vi "Overlay.vi"(8 "error in (no error)":errorcluster, 10 "Image In":T1, 11 "Overlay Base in":refnum<class "Analyze Results SHG-AK.lvclass">) -> (0 "error out":errorcluster, 2 "Image out":T1, 3 "Overlay Base out":refnum<class "Analyze Results SHG-AK.lvclass">)   [LabVIEW 2020, in "Analyze Results SHG-AK.lvclass"]
uses:
  Analyze Results SHG-AK.lvclass
  C:/POLARIS Programme/POLARIS-AS-3-Cams/Submodules/HIJ Vision/Analyze/Results and Overlays/Results Base/Analyze Results Base.lvclass
  <vilib>/vision/Image Controls.llb/IMAQ Image.ctl
  Results Base/Analyze Results Base.lvclass/Analyze Results Base.ctl
  Analyze Results SHG-AK.lvclass/Analyze Results SHG-AK.ctl
  Results Base/Read Overlay_.vi
  Results Base/Read Overlay colors.vi
  Results Base/Read Font, Size & Style.vi
  Results Base/Read Position.vi
  Read FWHM .vi
  Read FWHM Gaussfit.vi
  Results Base/Analyze Results Base.lvclass
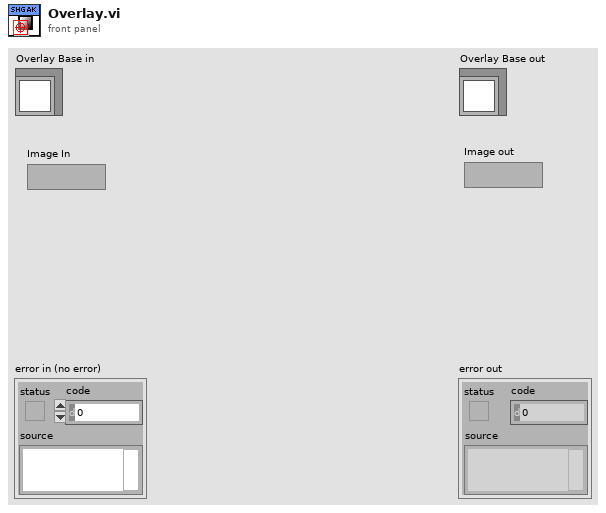
[diagram p1: front panel]
types:
  T1 = typedef "IMAQ Image.ctl" = refnum<image>
  T2 = cluster{"Desired Font (Application)":enum16{"User-specified Font", "Application Font", "System Font", "Dialog Font"}, "[User-specified Font]":cluster{"Font Name":string, "Size":i16, "Strikeout?":bool, "Italic?":bool, "Underline?":bool, "Outline?":bool, "Shadow?":bool, "Bold?":bool, "Rotation Angle":dbl}, "Horizontal Alignment":i16, "Vertical Alignment":i16}
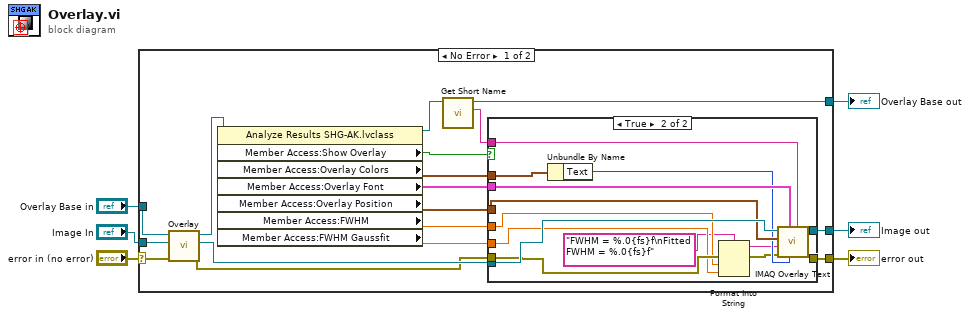
[diagram p0: block diagram]
diagram:
  n1 = case shown="No Error" "error in (no error)" {
    selector: "error in (no error)" -> [w10 w42]
    tunnel: "Image In" -> [w22 w41]
    tunnel: "Overlay Base in" -> [w21 w40]
    tunnel: [w8 w40] -> w4
    tunnel: [w17 w41] -> w3
    tunnel: [w16 w42] -> w2
    frame No Error {
      n2 = call-parent "Overlay.vi"("error in (no error)"=w10, "Image In"=w22, "Overlay Base in"=w21) -> ("error out"=w15:errorcluster, "Image out"=w18:T1, "Overlay Base out"=w23:refnum<class "Analyze Results SHG-AK.lvclass">)  [unwired: 6 in]
      n3 = property class="Analyze Results SHG-AK.lvclass"(reference=w23) -> (reference out=w20:refnum<class "Analyze Results SHG-AK.lvclass">, "Member Access:Show Overlay"=w9:bool, "Member Access:Overlay Colors"=w19:cluster{"Border":u32, "Text":u32}, "Member Access:Overlay Font"=w11:T2, "Member Access:Overlay Position"=w14:cluster{"x":i16, "y":i16}, "Member Access:FWHM "=w13:dbl[unit], "Member Access:FWHM Gaussfit"=w12:dbl[unit])  [unwired: 1 in, 1 out]
      n4 = call-dynamic "Get Short Name.vi"("Analyze Results Base in"=w20) -> ("Short Name"=w7:string, "Analyze Results Base out"=w8:refnum<class "Analyze Results SHG-AK.lvclass">)  [unwired: 8 in, 1 out]
      n5 = case shown="True" w9 {
        tunnel: w19 -> [_ w39]
        tunnel: w18 -> [w25 w38]
        tunnel: [w25 w37] -> w17
        tunnel: [w24 w36] -> w16
        tunnel: w15 -> [w24 w35]
        tunnel: w14 -> [_ w34]
        tunnel: w13 -> [_ w33]
        tunnel: w12 -> [_ w32]
        tunnel: w11 -> [_ w31]
        tunnel: w7 -> [_ w30]
        frame False {
        }
        frame True {
          n6 = Unbundle By Name(w39) -> ("Text"=w29:u32)
          n7 = Format Into String(format string="FWHM = %.0{fs}f\nFitted FWHM = %.0{fs}f", error in=w35, w33, w32) -> (resulting string=w28:string, error out=w27:errorcluster)  [unwired: 1 in]
          n8 = call "IMAQ Overlay Text"("Group"=w30, "Text Color (black)"=w29, "Font, Size & Style"=w31, "error in (no error)"=w27, "String"=w28, "Origin"=w34, "Image"=w38) -> ("error out"=w36:errorcluster, "Image Out"=w37:T1)  [unwired: 3 in]
        }
      }
    }
    frame Error {
    }
  }
  "error out" <- w2
  "Overlay Base out" <- w4
  "Image out" <- w3
